vi "Работа с путем файла.vi"() -> ()   [LabVIEW 2021]
uses:
  CSVtxtcluster.ctl
panel:
  out "record(s)":T1[](array[typedef]) {"Knob" scale=0.0..10.0}
  in  "Cluster":T1 {"Knob" scale=0.0..10.0}
  in  "Knob":dbl(knob) scale=0.0..10.0
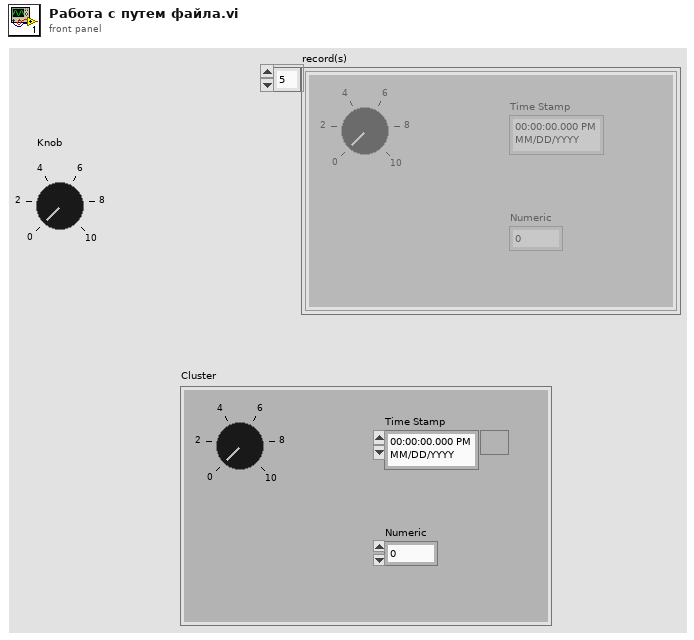
[diagram p1: front panel]
types:
  T1 = typedef "CSVtxtcluster.ctl" = cluster{"Knob":dbl, "Time Stamp":timestamp, "Numeric":dbl}
  T2 = enum16{"open", "replace", "create", "open or create", "replace or create", "replace or create with confirmation"}
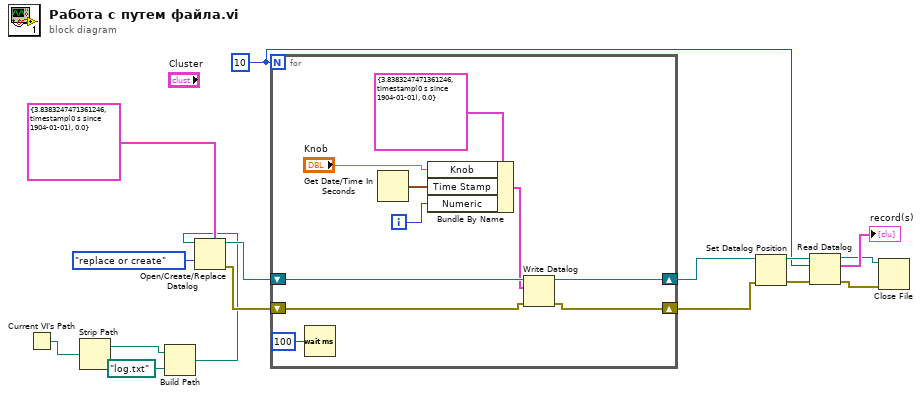
[diagram p0: block diagram]
diagram:
  w7 = 10
  n1 = Current VI's Path() -> (path=w1:path)
  n2 = Strip Path(path=w1) -> (stripped path=w4:path)  [unwired: 1 out]
  n3 = Build Path(base path=w4, name or relative path=path "log.txt") -> (appended path=w2:path)
  n4 = Open/Create/Replace Datalog(5:T1 {"Knob"=3.8383247471361246, "Time Stamp"=timestamp(0 s since 1904-01-01), "Numeric"=0.0} ("Cluster"), 10:T2."replace or create" ("operation (0:open)"), 11:w2) -> (0:w16:errorcluster, 3:w15:refnum<k1>)  [unwired: 3 in, 1 out]
  n5 = for {
    N: w7 -> [_]
    shift-right: [w25] -> w8
    shift-left: w16 -> [w24]
    shift-right: [w19] -> w10
    shift-left: w15 -> [w18]
    i -> [w22]
    n6 = Wait (ms)(milliseconds to wait=u32 100) -> ()  [unwired: 1 out]
    n7 = Get Date/Time In Seconds() -> (seconds since 1Jan1904=w21:timestamp)
    n8 = Bundle By Name(cluster=T1 {"Knob"=3.8383247471361246, "Time Stamp"=timestamp(0 s since 1904-01-01), "Numeric"=0.0} ("Cluster"), "Knob"="Knob", "Time Stamp"=w21, "Numeric"=w22) -> (w17:T1)
    n9 = Write Datalog(4:w24, 6:w17, 7:w18) -> (0:w25:errorcluster, 3:w19:refnum<k1>)
  }
  n10 = Set Datalog Position(4:w8, 7:w10) -> (0:w11:errorcluster, 3:w9:refnum<k1>)  [unwired: 2 in]
  n11 = Read Datalog(4:w11, 6:w7, 7:w9) -> (0:w6:errorcluster, 2:→"record(s)":T1[], 3:w5:refnum<k1>)
  n12 = Close File(refnum=w5, error in=w6) -> ()  [unwired: 2 out]
